vi "GenerateListOfCoordintes (SubVI).vi"(0 "Module side length [mm]":dbl=97.54, 1 "Nloops":i32=1, 2 "A [mm]":cluster{"X":dbl, "Y":dbl, "Z":dbl}={"X"=-61.753, "Y"=-124.535, "Z"=-0.811426}, 3 "x to fiducial [um]":dbl=460.0, 4 "y to fiducial [um]":dbl=1060.0) -> (7 "Generated List of Module Coordinates":dbl[][](array[numeric]))   [LabVIEW 2016]
panel:
  out "D [mm]":cluster{"X":dbl, "Y":dbl, "Z":dbl}={"X"=-61.753, "Y"=-124.535, "Z"=-0.811426}
  out "C [mm]":cluster{"X":dbl, "Y":dbl, "Z":dbl}={"X"=-61.753, "Y"=-124.535, "Z"=-0.811426}
  out "B [mm]":cluster{"X":dbl, "Y":dbl, "Z":dbl}={"X"=-61.753, "Y"=-124.535, "Z"=-0.811426}
  out "lv [mm]":dbl
  out "lh [mm]":dbl
  # "2*230 um for 4dots"
  # "2*(230+300+500) um for 4dots"
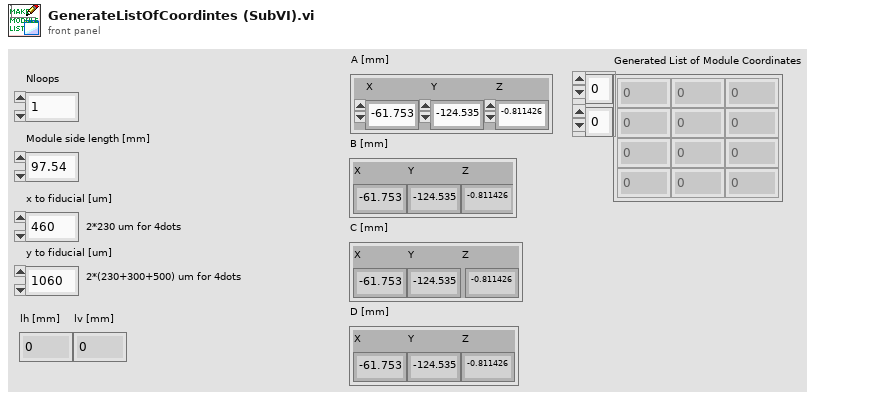
[diagram p1: front panel]
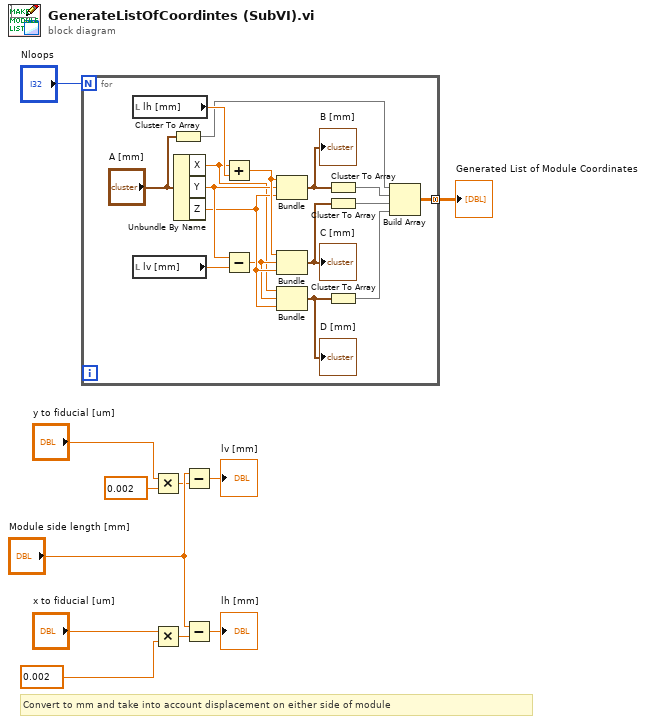
[diagram p0: block diagram]
diagram:
  # "Convert to mm and take into account displacement on either side of module"
  n1 = for {
    N: "Nloops" -> [_]
    tunnel: [w12] -> w1 mode=concatenating
    n2 = local read "lh [mm]"() -> (w27:dbl)
    n3 = local read "lv [mm]"() -> (w24:dbl)
    n4 = Cluster To Array(cluster="A [mm]") -> (array=w19:dbl[])
    n5 = Unbundle By Name("A [mm]") -> ("X"=w21:dbl, "Y"=w25:dbl, "Z"=w23:dbl)
    n6 = Add(x=w21, y=w27) -> (x+y=w26:dbl)
    n7 = Subtract(x=w25, y=w24) -> (x-y=w22:dbl)
    n8 = Bundle(w26, "Y"=w25, "Z"=w23) -> (w18:cluster{dbl, "Y":dbl, "Z":dbl})  [unwired: 1 in]
    "B [mm]" <- w18
    n9 = Bundle(w26, w22, "Z"=w23) -> (w17:cluster{dbl, dbl, "Z":dbl})  [unwired: 1 in]
    "C [mm]" <- w17
    n10 = Bundle("X"=w21, w22, "Z"=w23) -> (w16:cluster{"X":dbl, dbl, "Z":dbl})  [unwired: 1 in]
    "D [mm]" <- w16
    n11 = Cluster To Array(cluster=w18) -> (array=w15:dbl[])
    n12 = Cluster To Array(cluster=w17) -> (array=w14:dbl[])
    n13 = Cluster To Array(cluster=w16) -> (array=w13:dbl[])
    n14 = Build Array(w19, w15, w14, w13) -> (w12:dbl[][])
  }
  "Generated List of Module Coordinates" <- w1
  n15 = Multiply(x="y to fiducial [um]", y=0.002) -> (x*y=w3:dbl)
  n16 = Multiply(x="x to fiducial [um]", y=0.002) -> (x*y=w6:dbl)
  n17 = Subtract(x="Module side length [mm]", y=w3) -> (x-y=→"lv [mm]":dbl)
  n18 = Subtract(x="Module side length [mm]", y=w6) -> (x-y=→"lh [mm]":dbl)
